vi "3d_display.vi"() -> ()   [LabVIEW 2009]
uses:
  <vilib>/Analysis/NI_AALBase.lvlib
panel:
  out "Acceleration Graph":dynamicdata(graph)=[{"t0"=timestamp(3349182606.852725 s since 1904-01-01), "dt"=9.999999999999999e-05, "Y"=array[1000 elements], "attributes"=variant("NI_ChannelName"=variant(string "x_accel"), "NI_UnitDescription"=variant(string "Volts"))}, {"t0"=timestamp(3349182606.852746 s since 1904-01-01), "dt"=9.999999999999999e-05, "Y"=array[1000 elements], "attributes"=variant("NI_ChannelName"=variant(string "y_accel"), "NI_UnitDescription"=variant(string "Volts"))}, {"t0"=timestamp(3349182606.8527665 s since 1904-01-01), "dt"=9.999999999999999e-05, "Y"=array[1000 elements], "attributes"=variant("NI_ChannelName"=variant(string "z_accel"), "NI_UnitDescription"=variant(string "Volts"))}]
  in  "stop":bool
  in  "x offset":dbl=1.25
  in  "x gain":dbl=5.0
  in  "y offset":dbl=1.25
  in  "y gain":dbl=5.0
  in  "z offset":dbl=1.25
  in  "z gain":dbl=5.0
  out "Velocity":dynamicdata(graph)=[{"t0"=timestamp(3349182606.852725 s since 1904-01-01), "dt"=9.999999999999999e-05, "Y"=array[1000 elements], "attributes"=variant("NI_ChannelName"=variant(string "x_accel (Integral (Sum[Xdt]))"), "NI_OriginalChannelName"=variant(string "x_accel"), "NI_UnitDescription"=variant(string "Volts"))}, {"t0"=timestamp(3349182606.852746 s since 1904-01-01), "dt"=9.999999999999999e-05, "Y"=array[1000 elements], "attributes"=variant("NI_ChannelName"=variant(string "y_accel (Integral (Sum[Xdt]))"), "NI_OriginalChannelName"=variant(string "y_accel"), "NI_UnitDescription"=variant(string "Volts"))}, {"t0"=timestamp(3349182606.8527665 s since 1904-01-01), "dt"=9.999999999999999e-05, "Y"=array[1000 elements], "attributes"=variant("NI_ChannelName"=variant(string "z_accel (Integral (Sum[Xdt]))"), "NI_OriginalChannelName"=variant(string "z_accel"), "NI_UnitDescription"=variant(string "Volts"))}] caption="Result"
  out "Position":dynamicdata(graph)=[{"t0"=timestamp(3349182606.852725 s since 1904-01-01), "dt"=9.999999999999999e-05, "Y"=array[1000 elements], "attributes"=variant("NI_ChannelName"=variant(string "x_accel (Integral (Sum[Xdt]))"), "NI_OriginalChannelName"=variant(string "x_accel"), "NI_UnitDescription"=variant(string "Volts"))}, {"t0"=timestamp(3349182606.852746 s since 1904-01-01), "dt"=9.999999999999999e-05, "Y"=array[1000 elements], "attributes"=variant("NI_ChannelName"=variant(string "y_accel (Integral (Sum[Xdt]))"), "NI_OriginalChannelName"=variant(string "y_accel"), "NI_UnitDescription"=variant(string "Volts"))}, {"t0"=timestamp(3349182606.8527665 s since 1904-01-01), "dt"=9.999999999999999e-05, "Y"=array[1000 elements], "attributes"=variant("NI_ChannelName"=variant(string "z_accel (Integral (Sum[Xdt]))"), "NI_OriginalChannelName"=variant(string "z_accel"), "NI_UnitDescription"=variant(string "Volts"))}] caption="Result"
  out "Z mean volts":dbl format="%0.4f"
  out "Z mean acceleration":dbl format="%0.4f"
  out "Y mean volts":dbl format="%0.4f"
  out "X mean volts":dbl format="%0.4f"
  out "Y mean acceleration":dbl format="%0.4f"
  out "X mean acceleration":dbl format="%0.4f"
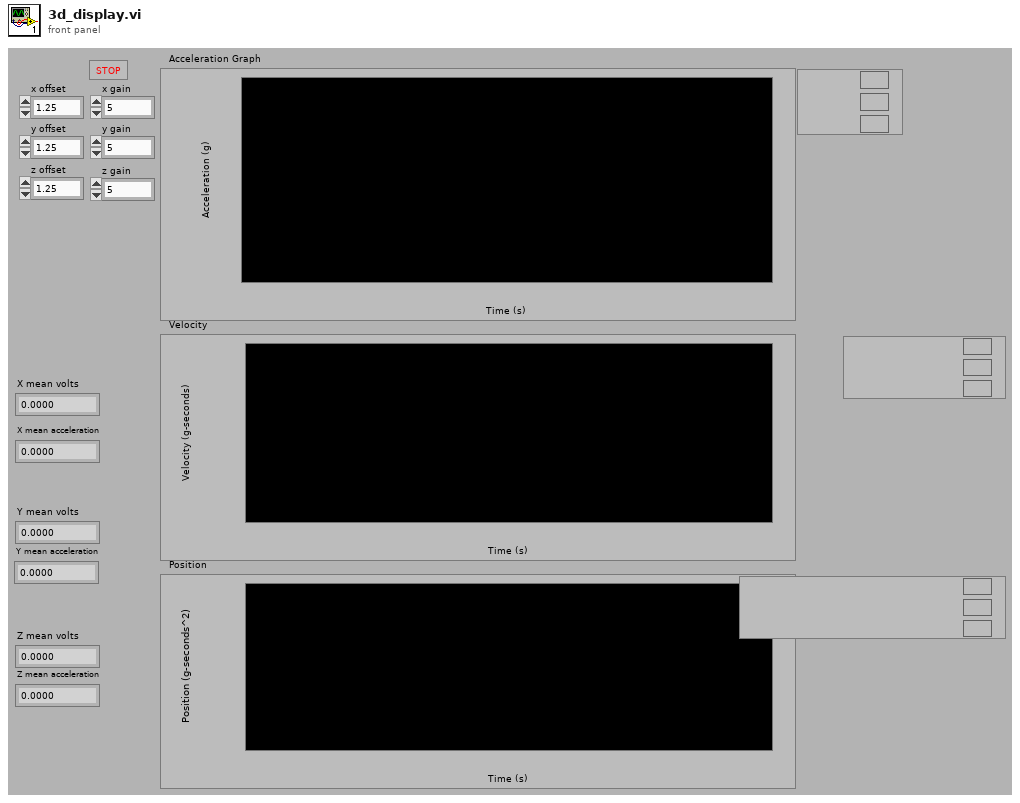
[diagram p1: front panel]
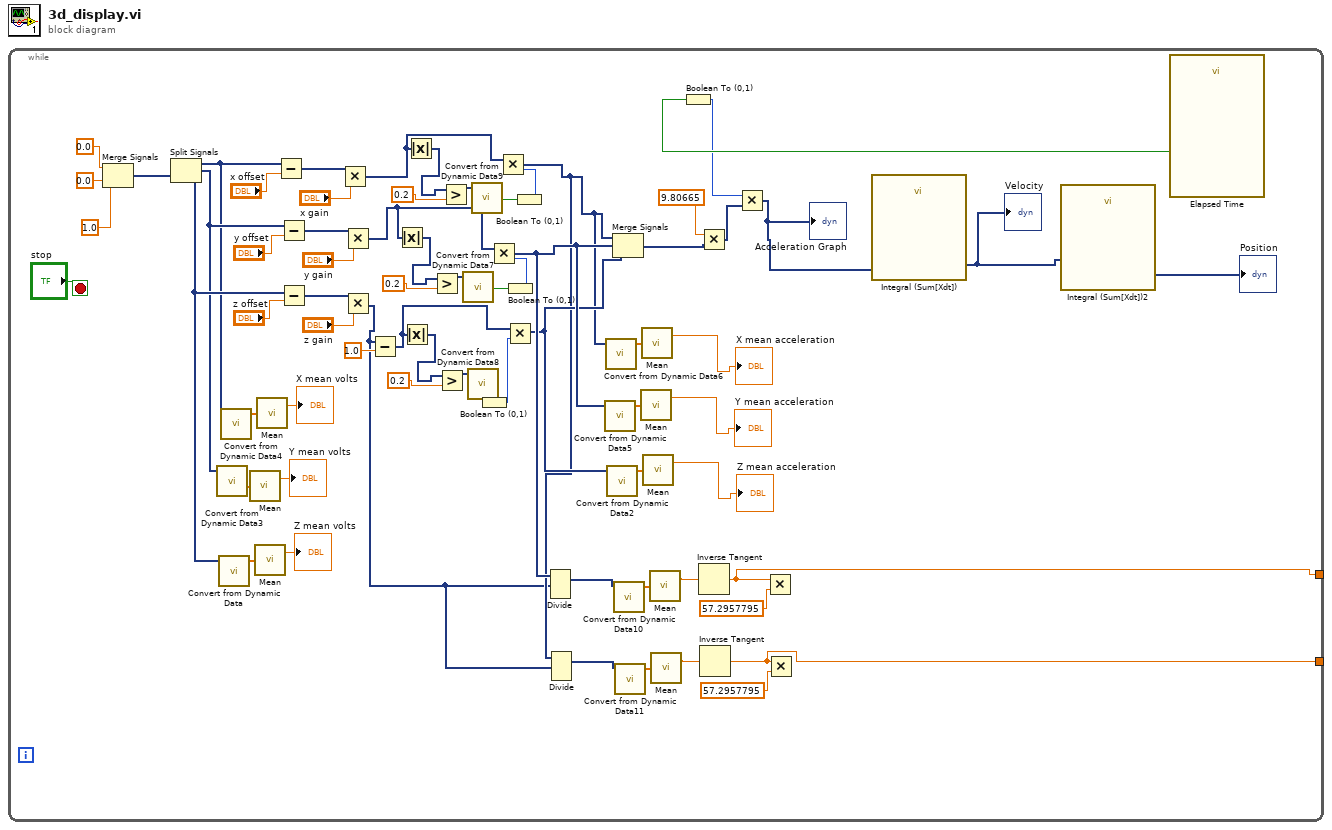
[diagram p0: block diagram]
diagram:
  n1 = while {
    tunnel: [w2] -> _
    tunnel: [w1] -> _
    stop <- "stop" stop-if-true
    n2 = Merge Signals(0.0, 0.0, 1.0) -> (w12:dynamicdata)
    n3 = Split Signals(w12) -> (w50:dynamicdata, w52:dynamicdata, w55:dynamicdata)  [unwired: 3 in]
    n4 = call "Convert from Dynamic Data3"("Dynamic Data Type"=w52) -> ("Array"=w51:dbl[])  [unwired: 3 in]
    n5 = call "Convert from Dynamic Data"("Dynamic Data Type"=w55) -> ("Array"=w59:dbl[])  [unwired: 3 in]
    n6 = call "Convert from Dynamic Data4"("Dynamic Data Type"=w50) -> ("Array"=w49:dbl[])  [unwired: 3 in]
    n7 = call <vilib>:"Mean.vi"("X"=w51) -> ("mean"=→"Y mean volts":dbl)  [unwired: 1 out]
    n8 = call <vilib>:"Mean.vi"("X"=w59) -> ("mean"=→"Z mean volts":dbl)  [unwired: 1 out]
    n9 = call <vilib>:"Mean.vi"("X"=w49) -> ("mean"=→"X mean volts":dbl)  [unwired: 1 out]
    n10 = Subtract(x=w50, y="x offset") -> (x-y=w69:dynamicdata)
    n11 = Subtract(x=w52, y="y offset") -> (x-y=w65:dynamicdata)
    n12 = Subtract(x=w55, y="z offset") -> (x-y=w44:dynamicdata)
    n13 = Multiply(x=w69, y="x gain") -> (x*y=w25:dynamicdata)
    n14 = Multiply(x=w65, y="y gain") -> (x*y=w43:dynamicdata)
    n15 = Multiply(x=w44, y="z gain") -> (x*y=w3:dynamicdata)
    n16 = Subtract(x=w3, y=1.0) -> (x-y=w31:dynamicdata)
    n17 = Absolute Value(x=w43) -> (abs(x)=w42:dynamicdata)
    n18 = Absolute Value(x=w31) -> (abs(x)=w37:dynamicdata)
    n19 = Absolute Value(x=w25) -> (abs(x)=w30:dynamicdata)
    n20 = Greater?(x=w42, y=0.2) -> (0:w39:dynamicdata)
    n21 = Greater?(x=w37, y=0.2) -> (0:w35:dynamicdata)
    n22 = Greater?(x=w30, y=0.2) -> (0:w27:dynamicdata)
    n23 = call "Convert from Dynamic Data7"("Dynamic Data Type"=w39) -> ("Scalar"=w38:bool)  [unwired: 3 in]
    n24 = call "Convert from Dynamic Data8"("Dynamic Data Type"=w35) -> ("Scalar"=w34:bool)  [unwired: 3 in]
    n25 = call "Convert from Dynamic Data9"("Dynamic Data Type"=w27) -> ("Scalar"=w26:bool)  [unwired: 3 in]
    n26 = Boolean To (0,1)(Boolean=w34) -> (0, 1=w33:i16)
    n27 = Boolean To (0,1)(Boolean=w38) -> (0, 1=w40:i16)
    n28 = Multiply(x=w43, y=w40) -> (x*y=w16:dynamicdata)
    n29 = Multiply(x=w31, y=w33) -> (x*y=w15:dynamicdata)
    n30 = Boolean To (0,1)(Boolean=w26) -> (0, 1=w28:i16)
    n31 = Multiply(x=w25, y=w28) -> (x*y=w4:dynamicdata)
    n32 = Divide(1:w3, 2:w16) -> (0:w18:dynamicdata)  [unwired: 1 in, 1 out]
    n33 = Divide(1:w3, 2:w4) -> (0:w6:dynamicdata)  [unwired: 1 in, 1 out]
    n34 = call "Convert from Dynamic Data5"("Dynamic Data Type"=w16) -> ("Array"=w46:dbl[])  [unwired: 3 in]
    n35 = call "Convert from Dynamic Data6"("Dynamic Data Type"=w4) -> ("Array"=w45:dbl[])  [unwired: 3 in]
    n36 = call "Convert from Dynamic Data2"("Dynamic Data Type"=w15) -> ("Array"=w58:dbl[])  [unwired: 3 in]
    n37 = Merge Signals(w4, w16, w15) -> (w56:dynamicdata)
    n38 = call "Convert from Dynamic Data10"("Dynamic Data Type"=w18) -> ("Array"=w20:dbl[])  [unwired: 3 in]
    n39 = call "Convert from Dynamic Data11"("Dynamic Data Type"=w6) -> ("Array"=w8:dbl[])  [unwired: 3 in]
    n40 = call <vilib>:"Mean.vi"("X"=w46) -> ("mean"=→"Y mean acceleration":dbl)  [unwired: 1 out]
    n41 = call <vilib>:"Mean.vi"("X"=w45) -> ("mean"=→"X mean acceleration":dbl)  [unwired: 1 out]
    n42 = call <vilib>:"Mean.vi"("X"=w58) -> ("mean"=→"Z mean acceleration":dbl)  [unwired: 1 out]
    n43 = call <vilib>:"Mean.vi"("X"=w20) -> ("mean"=w19:dbl)  [unwired: 1 out]
    n44 = call <vilib>:"Mean.vi"("X"=w8) -> ("mean"=w7:dbl)  [unwired: 1 out]
    n45 = Multiply(x=9.80665, y=w56) -> (x*y=w22:dynamicdata)
    n46 = Inverse Tangent(1:w19) -> (0:w2:dbl)
    n47 = Inverse Tangent(1:w7) -> (0:w1:dbl)
    n48 = Multiply(x=w2, y=57.2957795) -> ()  [unwired: 1 out]
    n49 = Multiply(x=w1, y=57.2957795) -> ()  [unwired: 1 out]
    n50 = call "Elapsed Time"() -> ("Time has Elapsed"=w24:bool)  [unwired: 12 in, 7 out]
    n51 = Boolean To (0,1)(Boolean=w24) -> (0, 1=w21:i16)
    n52 = Multiply(x=w21, y=w22) -> (x*y=w23:dynamicdata)
    "Acceleration Graph" <- w23
    n53 = call "Integral (Sum[Xdt])"("Signals"=w23) -> ("Result"=w14:dynamicdata)  [unwired: 5 in, 1 out]
    "Velocity" <- w14
    n54 = call "Integral (Sum[Xdt])2"("Signals"=w14) -> ("Result"=→"Position":dynamicdata)  [unwired: 5 in, 1 out]
  }
